vi "Parse XSDVersion.vi"(8 "error in":errorcluster, 11 "Node In":refnum<k20>) -> (0 "error out":errorcluster, 2 "XSDVersion":T1, 3 "Node Out":refnum<k20>)   [LabVIEW 2024, in "Parser.lvlib" / "Custom Device Config.lvclass"]
uses:
  Custom Device Config.lvclass
  Parser.lvlib
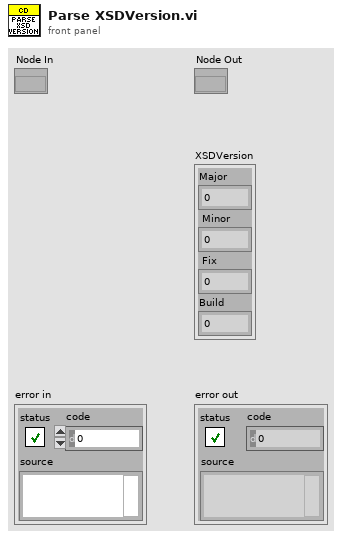
[diagram p1: front panel]
types:
  T1 = cluster{"Major":u32, " Minor":u32, " Fix":u32, "Build":u32}
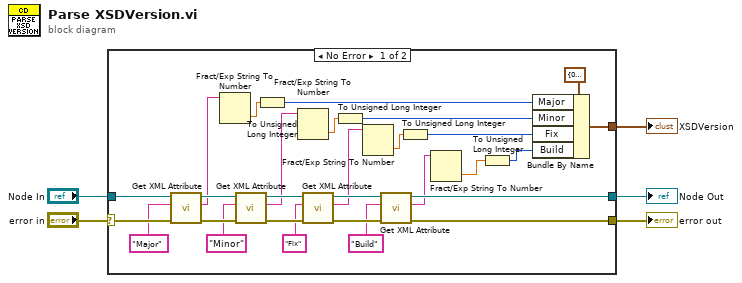
[diagram p0: block diagram]
diagram:
  n1 = case shown="No Error" "error in" {
    selector: "error in" -> [w32 w35]
    tunnel: [w33 w35] -> w4
    tunnel: [w24 w34] -> w3
    tunnel: "Node In" -> [w28 w34]
    tunnel: [w18 _] -> w1
    frame No Error {
      n2 = call "Get XML Attribute.vi"("error in"=w32, "Attribute Name"="Major", "XML Node"=w28) -> ("error out"=w31:errorcluster, "Attribute Value"=w16:string, "XML Node out"=w27:refnum<k20>)  [unwired: 6 in]
      n3 = Fract/Exp String To Number(string=w16) -> (number=w17:dbl)  [unwired: 3 in, 1 out]
      n4 = call "Get XML Attribute.vi"("error in"=w31, "Attribute Name"="Minor", "XML Node"=w27) -> ("error out"=w30:errorcluster, "Attribute Value"=w11:string, "XML Node out"=w26:refnum<k20>)  [unwired: 6 in]
      n5 = To Unsigned Long Integer(number=w17) -> (unsigned 32bit integer=w15:u32)
      n6 = Fract/Exp String To Number(string=w11) -> (number=w14:dbl)  [unwired: 3 in, 1 out]
      n7 = call "Get XML Attribute.vi"("error in"=w30, "Attribute Name"="Fix", "XML Node"=w26) -> ("error out"=w29:errorcluster, "Attribute Value"=w9:string, "XML Node out"=w25:refnum<k20>)  [unwired: 6 in]
      n8 = To Unsigned Long Integer(number=w14) -> (unsigned 32bit integer=w12:u32)
      n9 = Fract/Exp String To Number(string=w9) -> (number=w13:dbl)  [unwired: 3 in, 1 out]
      n10 = call "Get XML Attribute.vi"("error in"=w29, "Attribute Name"="Build", "XML Node"=w25) -> ("error out"=w33:errorcluster, "Attribute Value"=w7:string, "XML Node out"=w24:refnum<k20>)  [unwired: 6 in]
      n11 = To Unsigned Long Integer(number=w13) -> (unsigned 32bit integer=w10:u32)
      n12 = Fract/Exp String To Number(string=w7) -> (number=w8:dbl)  [unwired: 3 in, 1 out]
      n13 = To Unsigned Long Integer(number=w8) -> (unsigned 32bit integer=w6:u32)
      n14 = Bundle By Name(cluster=T1 {"Major"=0, " Minor"=0, " Fix"=0, "Build"=0} ("XSDVersion"), "Major"=w15, "Minor"=w12, "Fix"=w10, "Build"=w6) -> (w18:T1)
    }
    frame Error {
    }
  }
  "XSDVersion" <- w1
  "Node Out" <- w3
  "error out" <- w4
